vi "test checksum.vi"() -> ()   [LabVIEW 2016]
uses:
  type defs/Pelco_D_cmd.vi
panel:
  out "CHKSUM":string
  out "rev CHKSUM":string
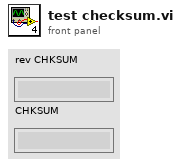
[diagram p1: front panel]
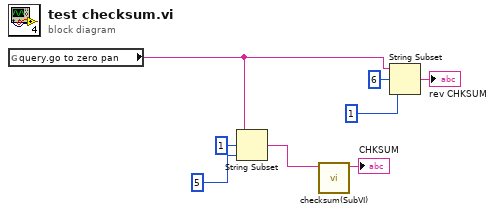
[diagram p0: block diagram]
diagram:
  n1 = global read "Pelco_D_cmd.vi" "query.go to zero pan"() -> (w1:string)
  n2 = String Subset(string=w1, offset (0)=1, length (rest)=5 ("length (rest)")) -> (substring=w6:string)
  n3 = call "checksum(SubVI).vi"("response"=w6) -> ("CHKSUM"=→"CHKSUM":string)  [unwired: 10 in]
  n4 = String Subset(string=w1, offset (0)=6, length (rest)=1 ("length (rest)")) -> (substring=→"rev CHKSUM":string)
